vi "Get PGSQL Info.vi"(8 "error in (no error)":errorcluster, 10 "Get PGSQL Info":string, 11 "Instrument.Temperhum in":refnum<class "Instrument.Temperhum.lvclass">) -> (0 "error out":errorcluster, 3 "Instrument.Temperhum out":refnum<class "Instrument.Temperhum.lvclass">)   [LabVIEW 2019, in "Instrument.Temperhum.lvclass"]
uses:
  Instrument.Temperhum.lvclass
  Typedefs/PublicEvents--Instrument.Temperhum.Get PGSQL Info.ctl
  Instrument.Temperhum.lvclass/Instrument.Temperhum.ctl
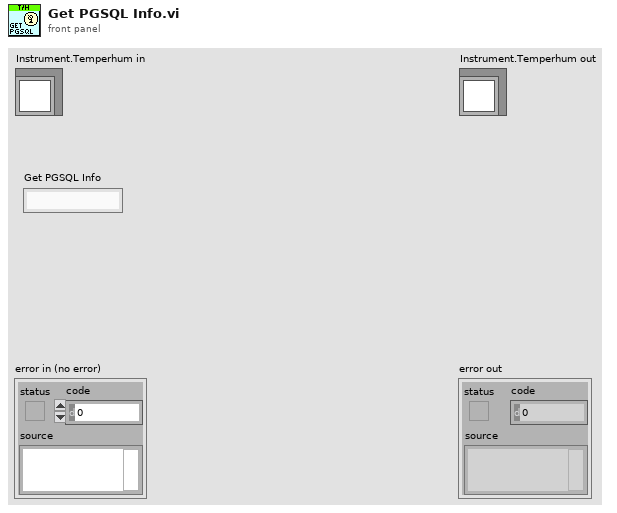
[diagram p1: front panel]
types:
  T1 = typedef "Instrument.Temperhum.lvclass/PublicEvents--Instrument.Temperhum.Get PGSQL Info.ctl" = string
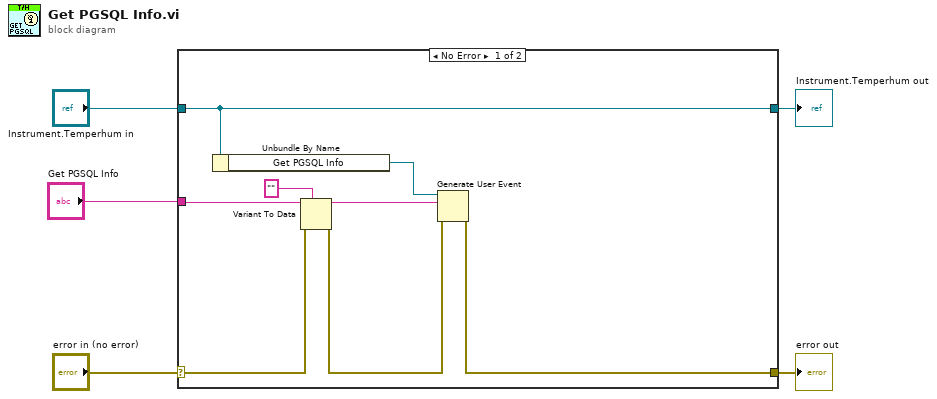
[diagram p0: block diagram]
diagram:
  n1 = case shown="No Error" "error in (no error)" {
    selector: "error in (no error)" -> [w7 w15]
    tunnel: [w11 w15] -> w4
    tunnel: [w13 w14] -> w2
    tunnel: "Instrument.Temperhum in" -> [w13 w14]
    tunnel: "Get PGSQL Info" -> [w10 _]
    frame No Error {
      n2 = Unbundle By Name(w13) -> ("Get PGSQL Info"=w12:refnum<user-event>)
      n3 = Variant To Data(error in=w7, type=T1 "" ("event data"), Variant=w10) -> (data=w8:T1, error out=w6:errorcluster)
      n4 = Generate User Event(user event=w12, event data cluster=w8, error in=w6) -> (error out=w11:errorcluster)  [unwired: 1 in, 1 out]
    }
    frame Error {
    }
  }
  "error out" <- w4
  "Instrument.Temperhum out" <- w2
